vi "WaitUntilRunning.vi"(8 "check interval (ms)":dbl) -> ()   [LabVIEW 2018]
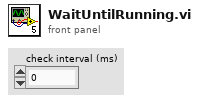
[diagram p1: front panel]
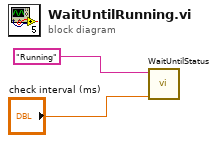
[diagram p0: block diagram]
diagram:
  n1 = call "WaitUntilStatus.vi"("check interval (ms)"="check interval (ms)", "target status"="Running") -> ()  [unwired: 10 in]
